vi "property_cursors_point_size_write.vi"(4 "error in (no error)":errorcluster, 5 "Value":dbl, 6 "Container State":T29, 7 "Display State In":T1) -> (0 "error out":errorcluster, 3 "Display State Out":T1)   [LabVIEW 2020, in "3DPC_SurfacePlot.xctl"]
uses:
  <vilib>/Native 3D Graph/xcontrol/3DPC_SurfacePlot.xctl
  <vilib>/_xctls/Container State.ctl
  <vilib>/Native 3D Graph/xcontrol/State.ctl
  <vilib>/Native 3D Graph/typedefs/prop_graph.ctl
  <vilib>/Native 3D Graph/typedefs/all_non_graph_prop.ctl
  <vilib>/Native 3D Graph/typedefs/prop_plot_all_array.ctl
  <vilib>/Native 3D Graph/typedefs/prop_plot_all.ctl
  <vilib>/Native 3D Graph/typedefs/prop_plot_projection.ctl
  <vilib>/Native 3D Graph/typedefs/prop_plot_surface.ctl
  <vilib>/Native 3D Graph/typedefs/prop_plot_contour.ctl
  <vilib>/Native 3D Graph/typedefs/prop_plot_normal.ctl
  <vilib>/Native 3D Graph/typedefs/prop_plot_point_line.ctl
  <vilib>/Native 3D Graph/typedefs/prop_value_pair_all.ctl
  <vilib>/Native 3D Graph/typedefs/prop_value_pair_1d.ctl
  <vilib>/Native 3D Graph/typedefs/prop_axes_all.ctl
  <vilib>/Native 3D Graph/typedefs/prop_axes_grid.ctl
  <vilib>/Native 3D Graph/typedefs/prop_axes_ticks.ctl
  <vilib>/Native 3D Graph/typedefs/range_cluster.ctl
  <vilib>/Native 3D Graph/typedefs/min_max.ctl
  <vilib>/Native 3D Graph/typedefs/prop_axes_captions.ctl
  <vilib>/Native 3D Graph/typedefs/prop_axes_labels.ctl
  <vilib>/Native 3D Graph/typedefs/prop_axes_autorange.ctl
  <vilib>/Native 3D Graph/typedefs/prop_cursor_all_array.ctl
  <vilib>/Native 3D Graph/typedefs/prop_cursor_point.ctl
  <vilib>/Native 3D Graph/typedefs/prop_cursor_position.ctl
  <vilib>/Native 3D Graph/typedefs/prop_cursor_line.ctl
  <vilib>/Native 3D Graph/typedefs/prop_cursor_plane.ctl
  <vilib>/Native 3D Graph/typedefs/prop_cursor_text.ctl
  <vilib>/Native 3D Graph/typedefs/prop_format.ctl
  <vilib>/Native 3D Graph/typedefs/prop_lighting.ctl
  <vilib>/_xctls/XControlSupport.lvlib
panel:
  # "Replace the Value Control below with a Control of desired type.\nDo not remove this Control or the others from the connector pane.\nDo not change the connector pane pattern.\nThe Value control should always be the third terminal from top on the input side in the connector pane."
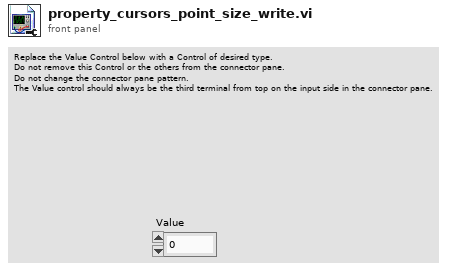
[diagram p1: front panel]
types:
  T1 = typedef "3DPC_SurfacePlot.xctl/State.ctl" = cluster{"Graph Properties":T2, "Plot/Axes/Cursor Properties":T3, "Active Plot":i32, "Active Axis":i32, "Active Cursor":i32, "Disable Updates":bool}
  T2 = typedef "3DPC_SurfacePlot.xctl/prop_graph.ctl" = cluster{"Projection Mode":enum16{"Orthographic", "Perspective"}, "View Direction":enum32{"Towards X-Y Plane", "Towards Y-Z Plane", "Towards X-Z Plane", "User Define"}, "Plot Area Color":u32, "Fast Draw":bool, "X-Y":bool, "Y-Z":bool, "X-Z":bool, "Lighting":bool, "Refnum Queue":refnum<queue>}
  T3 = typedef "3DPC_SurfacePlot.xctl/all_non_graph_prop.ctl" = cluster{"Plot Properties Array":T4, "Value Pair Properties":T11, "Axes Properties":T13, "Cursor Properties Array":T21, "Format strings":T27, "Lighting Properties":T28, "Lights":cluster{"Position":cluster{"X":sgl, "Y":sgl, "Z":sgl}, "Direction":cluster{"X":sgl, "Y":sgl, "Z":sgl}}[]}
  T4 = typedef "3DPC_SurfacePlot.xctl/prop_plot_all_array.ctl" = T5[]
  T5 = typedef "3DPC_SurfacePlot.xctl/prop_plot_all.ctl" = cluster{"Projection Properties":T6, "Surface Properties":T7, "Contour Properties":T8, "Normal Properties":T9, "Points/Lines Properties":T10, "Plot ID":i32, "Coordinate System":enum16{"Cartesian", "Cylindrical", "Spherical"}}
  T6 = typedef "3DPC_SurfacePlot.xctl/prop_plot_projection.ctl" = cluster{"Draw XY":bool, "Draw YZ":bool, "Draw XZ":bool}
  T7 = typedef "3DPC_SurfacePlot.xctl/prop_plot_surface.ctl" = cluster{"Draw surface":bool, "Opacity":dbl, "Shading":bool, "Specular":i32, "Color Map":cluster{dbl, u32}[], "Interpolate Color":bool, "Absolute Colormap":bool}
  T8 = typedef "3DPC_SurfacePlot.xctl/prop_plot_contour.ctl" = cluster{"Contour color":u32, "Axis":enum16{"X", "Y", "Z"}, "Draw contour":bool, "Antialias":bool, "Line Width":sgl, "Contour Line Style":enum16{"Solid", "Dash", "Dot", "Dash Dot"}, "Mode":enum16{"Levels", "Intervals", "Level List"}, "Levels":sgl, "Intervals":sgl, "Anchored At":sgl, "Anchored":bool, "Level List":dbl[]}
  T9 = typedef "3DPC_SurfacePlot.xctl/prop_plot_normal.ctl" = cluster{"Normal color":u32, "Normal Length":sgl, "Normal Width":sgl, "Draw Normal":bool, "Antialiasing":bool}
  T10 = typedef "3DPC_SurfacePlot.xctl/prop_plot_point_line.ctl" = cluster{"Color":u32, "Antialiasing":bool, "Point Size":sgl, "Points / Lines":enum16{"None", "Points", "Lines", "Both"}, "Point Style":enum16{"Point", "EmptySquare", "Asterisk", "Diamond", "EmptyCircle", "Circle", "X"}, "Line Style":enum16{"Solid", "Dash", "Dot", "Dash Dot"}, "Line Width":sgl}
  T11 = typedef "3DPC_SurfacePlot.xctl/prop_value_pair_all.ctl" = cluster{"X Value Pairs":cluster{"Data Array":cluster{"Value":sgl, "Index":i32, "Name":string}[], "Show ticks":bool, "Show grid lines":bool, "Labels":enum16{"Value", "None", "Name"}}, "Y Value Pairs":T12, "Z Value Pairs":T12}
  T12 = typedef "3DPC_SurfacePlot.xctl/prop_value_pair_1d.ctl" = cluster{"Data Array":cluster{"Value":sgl, "Index":i32, "Name":string}[], "Show ticks":bool, "Show grid lines":bool, "Labels":enum16{"Value", "None", "Name"}}
  T13 = typedef "3DPC_SurfacePlot.xctl/prop_axes_all.ctl" = cluster{"Grid  Properties":T14, "Ticks Properties":T15, "from/to cluster":T16, "Caption Properties":T18, "Labels Properties":T19, "Auto Range On":T20}
  T14 = typedef "3DPC_SurfacePlot.xctl/prop_axes_grid.ctl" = cluster{"Grid Visible":cluster{"Draw X-grid":bool, "Draw Y-grid":bool, "Draw Z-grid":bool}, "Grid Color":cluster{"Color X":u32, "Color Y":u32, "Color Z":u32}}
  T15 = typedef "3DPC_SurfacePlot.xctl/prop_axes_ticks.ctl" = cluster{"Minor Count":cluster{"X":i32, "Y":i32, "Z":i32}, "Major Count":cluster{"X":i32, "Y":i32, "Z":i32}, "Major Ticks Visible":cluster{"X":bool, "Y":bool, "Z":bool}, "Minor Ticks Visible":cluster{"X":bool, "Y":bool, "Z":bool}, "Tick Color":cluster{"Color X":u32, "Color Y":u32, "Color Z":u32}}
  T16 = typedef "3DPC_SurfacePlot.xctl/range_cluster.ctl" = cluster{"X":T17, "Y":T17, "Z":T17, "Amplitude":T17}
  T17 = typedef "3DPC_SurfacePlot.xctl/min_max.ctl" = cluster{"Min":sgl, "Max":sgl}
  T18 = typedef "3DPC_SurfacePlot.xctl/prop_axes_captions.ctl" = cluster{"Show Captions":cluster{"Show X Caption":bool, "Show Z Caption":bool, "Show Y Caption":bool, "Show Opposite X Caption":bool, "Show Opposite Y Caption":bool, "Show Opposite Z Caption":bool}, "Captions":cluster{"Caption X":string, "Caption Y":string, "Caption Z":string}, "Caption Color":cluster{"Color X":u32, "Color Y":u32, "Color Z":u32}, "Caption Font Size":cluster{"Font Size X":i16, "Font Size Y":i16, "Font Size Z":i16}}
  T19 = typedef "3DPC_SurfacePlot.xctl/prop_axes_labels.ctl" = cluster{"Label Visible":cluster{"Show X Labels":bool, "Show Y Labels":bool, "Show Z Labels":bool, "Show Opposite X Labels":bool, "Show Opposite Y Labels":bool, "Show Opposite Z Labels":bool}, "Label Color":cluster{"Color X":u32, "Color Y":u32, "Color Z":u32}, "Label Font Size":cluster{"Font Size X":i16, "Font Size Y":i16, "Font Size Z":i16}}
  T20 = typedef "3DPC_SurfacePlot.xctl/prop_axes_autorange.ctl" = cluster{"X":bool, "Y":bool, "Z":bool}
  T21 = typedef "3DPC_SurfacePlot.xctl/prop_cursor_all_array.ctl" = cluster{"Cursor Visible":bool, "Cursor Enable":bool, "Cursor Point":T22, "Cursor Position":T23, "Cursor Line":T24, "Cursor Plane":T25, "Cursor Name":string, "Cursor Text":T26}[]
  T22 = typedef "3DPC_SurfacePlot.xctl/prop_cursor_point.ctl" = cluster{"Point Color":u32, "Point Size":dbl, "Point Visible":bool}
  T23 = typedef "3DPC_SurfacePlot.xctl/prop_cursor_position.ctl" = cluster{"Position X":dbl, "Position Y":dbl, "Position Z":dbl, "Position Snap To":enum16{"Fixed", "Nearest Plot", "Snap to Plot"}, "Polsition Pick Plot":u16, "Position Column":i32, "Position Row":i32}
  T24 = typedef "3DPC_SurfacePlot.xctl/prop_cursor_line.ctl" = cluster{"Line Color":u32, "Line Width":dbl, "Line Visible":bool}
  T25 = typedef "3DPC_SurfacePlot.xctl/prop_cursor_plane.ctl" = cluster{"Plane Opacity":dbl, "Plane Color":u32, "Plane YZ":bool, "Plane XZ":bool, "Plane XY":bool}
  T26 = typedef "3DPC_SurfacePlot.xctl/prop_cursor_text.ctl" = cluster{"Cursor Name":string, "Font Size":i32, "Show Position":bool, "Show Name":bool, "Text Color":u32, "Back Color":u32, "Opacity":dbl}
  T27 = typedef "3DPC_SurfacePlot.xctl/prop_format.ctl" = cluster{"XAxis":string, "YAxis":string, "ZAxis":string}
  T28 = typedef "3DPC_SurfacePlot.xctl/prop_lighting.ctl" = cluster{"Brightness":i32, "Focus":dbl, "Linear Attenuation":dbl, "Quadratic Attenuation":dbl}
  T29 = typedef "XControlSupport.lvlib/Container State.ctl" = cluster{"Indicator?":bool, "Run Mode?":bool, " Refnum":refnum<vi>}
  T30 = cluster{"Cursor Visible":bool, "Cursor Enable":bool, "Cursor Point":T22, "Cursor Position":T23, "Cursor Line":T24, "Cursor Plane":T25, "Cursor Name":string, "Cursor Text":T26}
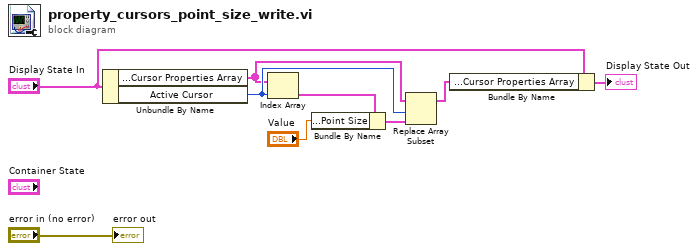
[diagram p0: block diagram]
diagram:
  n1 = Unbundle By Name("Display State In") -> ("Plot/Axes/Cursor Properties.Cursor Properties Array"=w4:T21, "Active Cursor"=w6:i32)
  n2 = Index Array(array=w4, index=w6) -> (element=w8:T30)
  n3 = Bundle By Name(cluster=w8, "Cursor Point.Point Size"="Value") -> (w5:T30)
  n4 = Replace Array Subset(array=w4, new element=w5, index=w6) -> (w3:T21)
  n5 = Bundle By Name(cluster="Display State In", "Plot/Axes/Cursor Properties.Cursor Properties Array"=w3) -> (→"Display State Out":T1)
  "error out" <- "error in (no error)"
